vi "Intake Motor Value.vi"(11 "Operator B Button":bool) -> ()   [LabVIEW 2019]
uses:
  .Team Code/Robot Global Data.vi
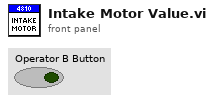
[diagram p1: front panel]
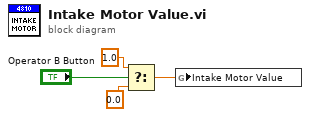
[diagram p0: block diagram]
diagram:
  n1 = Select(t=1.0, s="Operator B Button", f=0.0) -> (s? t:f=w1:dbl)
  n2 = global write "Robot Global Data.vi" "Intake Motor Value"(w1) -> ()
